vi "RunExperiment2.vi"(0 "object in":refnum<class "Application.lvclass">, 5 "error in (no error)":errorcluster) -> (14 "object out":refnum<class "Application.lvclass">, 15 "Average FPS":dbl, 16 "Waveform Graph":dbl[](graph), 17 "Finished":bool, 19 "error out":errorcluster)   [LabVIEW 2024, in "Application.lvclass"]
uses:
  Application.lvclass
  ExperimentSeries2_class/ExperimentSeries2.lvclass
  Experiment2_class/Experiment2.lvclass
  AD2_SDK_class/AD2_SDK.lvclass
  Hamamatsu_class/Hamamatsu.lvclass
  Application.lvclass/Application.ctl
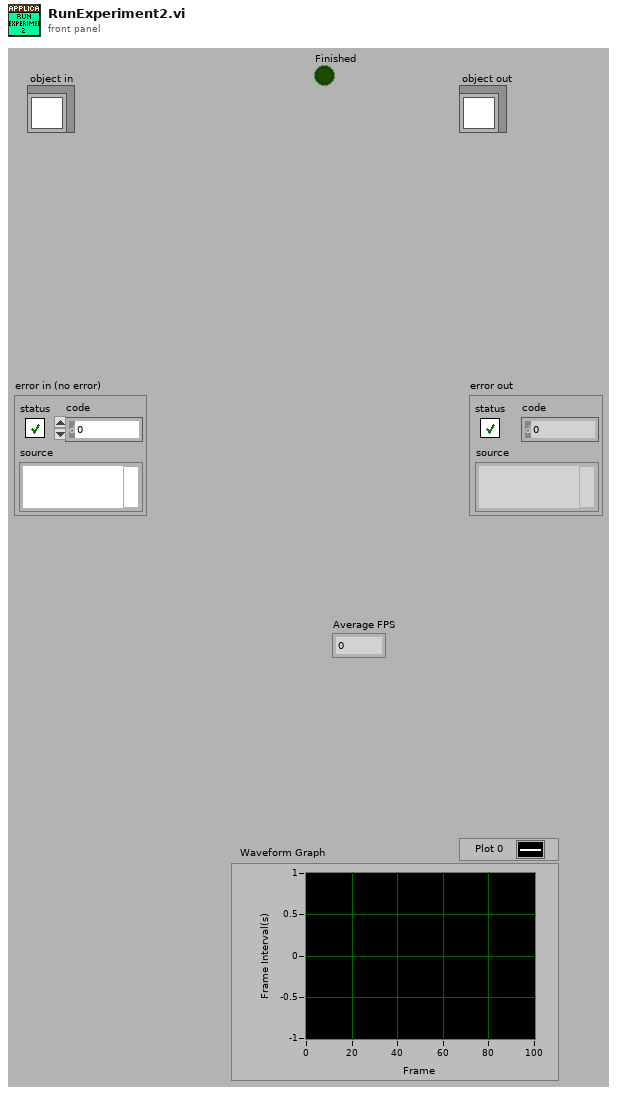
[diagram p1: front panel]
types:
  T1 = typedef "AD2_WFG_SDK.lvclass/WFG.ctl" = cluster{"Running":bool, "Ch1":T2, "Ch2":T2, "SyncronizeState":enum16{"Independent", "Ch1Master", "Ch2Master"}}
  T2 = typedef "AD2_WFG_SDK.lvclass/WFGCh.ctl" = cluster{"idxChannel":i32, "Settings out of range":bool, "Carrier":cluster{"Frequency (Hz)":dbl, "Amplitude (V)":dbl, "Offset(V)":dbl, "Symmetry(%) ":dbl, "Phase(Deg)":dbl, "Function":u16, "Enable":bool}, "Trigger":cluster{"secRun(0=Cont)":dbl, "secWait":dbl, "cRepeat(0=inf)":i32, "Repeat Trigger":bool, "TrigrSrc":T3}, "FM Mod":cluster{"Frequency (Hz)":dbl, "Amplitude (%)":dbl, "Offset(V)":dbl, "Symmetry(%) ":dbl, "Phase(Deg)":dbl, "Function 2":u16, "Enable":bool}}
  T3 = typedef "AD2_SDK.lvclass/AD2TriggerSources.ctl" = enum8{"trigrsrcNone", "trigsrcPC", "trigsrcDetectorAnalogIn", "trigsrcDetectorDigitalIn", "trigsrcAnalogIn", "trigsrcDigitalIn", "trigsrcDigitalOut", "trigsrcAnalogOut1", "trigsrcAnalogOut2", "trigsrcAnalogOut3", "trigsrcAnalogOut4", "trigsrcExternal1", "trigsrcExternal2", "trigsrcExternal3", "trigsrcExternal4", ""}
  T4 = typedef "AD2_DO_SDK.lvclass/DOTrigger.ctl" = cluster{"secRun(0=Cont)":dbl, "secWait":dbl, "cRepeat(0=inf)":i32, "Repeat Trigger":bool, "TrigrSrc":T3}
  T5 = cluster{"DO Trigger":T4, "ClockSettings":cluster{"Frequency":dbl, "Enable":bool, "IdleState":enum16{"Initial", "Low", "High", "Z"}}[]}
  T6 = cluster{"Frequency":dbl, "Enable":bool, "IdleState":enum16{"Initial", "Low", "High", "Z"}}[]
  T7 = cluster{"Master Pulse Settings":cluster{"Mode":u32, "Source":u32, "Interval":dbl, "Burst":u32}, "Capture mode":i32, "Frames":i32, "Dcam Trigger Source":i32, "External Options":cluster{"Polarity":i32, "Delay":dbl}, "ExposureTime(ms)":dbl}
  T8 = cluster{"Flush Flowrate":dbl, "flush volume (ul)":dbl, "WaitAfterFlush":dbl}
  T9 = typedef "Hamamatsu.lvclass/SubRegionLimits.ctl" = cluster{"H Offset":cluster{"Value":i32, "Limits":T10}, "V Offset":cluster{"Value":i32, "Limits":T10}, "H Size":cluster{"Value":i32, "Limits":T10}, "V Size":cluster{"Value":i32, "Limits":T10}}
  T10 = typedef "LVMinMaxIncTypeDef.ctl" = cluster{"Minimum":dbl, "Maximum":dbl, "Increment":dbl}
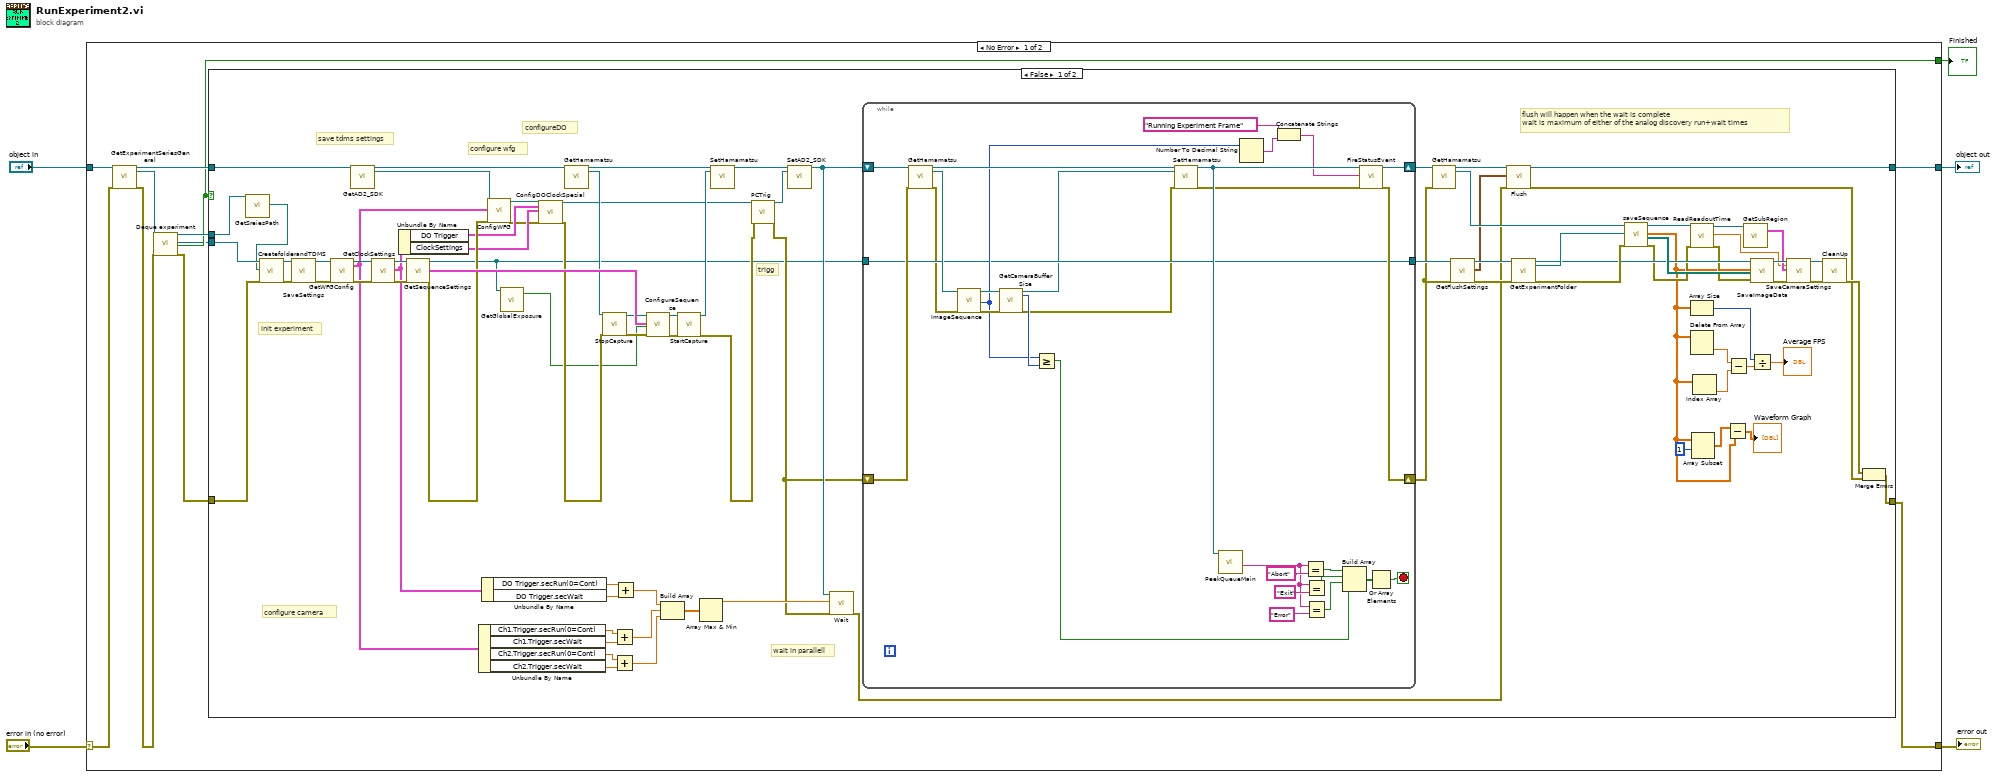
[diagram p0: block diagram]
diagram:
  n1 = case shown="No Error" "error in (no error)" {
    selector: "error in (no error)" -> [w12 w135]
    tunnel: [w8 w135] -> w4
    tunnel: [w16 w134] -> w2
    tunnel: "object in" -> [w15 w134]
    tunnel: [w7 _] -> w1
    frame No Error {
      n2 = call-dynamic "GetExperimentSeriesGeneral.vi"("object in"=w15, "error in (no error)"=w12) -> ("object out"=w14:refnum<class "Application.lvclass">, "ExperimentSeriesGeneral"=w13:refnum<class "ExperimentSeries2.lvclass">, "error out"=w11:errorcluster)  [unwired: 15 in]
      n3 = call-dynamic "Deque experiment.vi"("object in"=w13, "error in (no error)"=w11) -> ("object out"=w10:refnum<class "ExperimentSeries2.lvclass">, "Experiment2"=w6:refnum<class "Experiment2.lvclass">, "timed out?"=w7:bool, "error out"=w9:errorcluster)  [unwired: 14 in]
      n4 = case shown="False" w7 {
        tunnel: [w60 w133] -> w16
        tunnel: w14 -> [w102 w133]
        tunnel: w9 -> [w88 w132]
        tunnel: w10 -> [w72 _]
        tunnel: [w74 w132] -> w8
        tunnel: w6 -> [w99 _]
        frame False {
          # "wait in parallell"
          # "flush will happen when the wait is complete\nwait is maximum of either of the analog discovery run+wait times"
          # "init experiment"
          # "save tdms settings"
          # "trigg"
          # "configureDO"
          # "configure wfg"
          # "configure camera"
          n5 = call-dynamic "GetSreiesPath.vi"("object in"=w72) -> ("SeriesPath"=w71:path)  [unwired: 16 in, 2 out]
          n6 = call "CreatefolderandTDMS.vi"("object in"=w99, "Experiment Series"=w71, "error in (no error)"=w88) -> ("object out"=w98:refnum<class "Experiment2.lvclass">, "error out"=w97:errorcluster)  [unwired: 15 in]
          n7 = call-dynamic "SaveSettings.vi"("object in"=w98, "error in (no error)"=w97) -> ("object out"=w96:refnum<class "Experiment2.lvclass">, "error out"=w95:errorcluster)  [unwired: 16 in]
          n8 = call-dynamic "GetWFGConfig.vi"("object in"=w96, "error in (no error)"=w95) -> ("object out"=w65:refnum<class "Experiment2.lvclass">, "WFGConfig"=w34:T1, "error out"=w67:errorcluster)  [unwired: 15 in]
          n9 = call-dynamic "GetAD2_SDK.vi"("object in"=w102) -> ("object out"=w100:refnum<class "Application.lvclass">, "AD2_SDK"=w101:refnum<class "AD2_SDK.lvclass">)  [unwired: 16 in, 1 out]
          n10 = call-dynamic "GetClockSettings.vi"("object in"=w65, "error in (no error)"=w67) -> ("object out"=w64:refnum<class "Experiment2.lvclass">, "DOClockSettings"=w19:T5, "error out"=w66:errorcluster)  [unwired: 15 in]
          n11 = Unbundle By Name(w19) -> ("DO Trigger"=w63:T4, "ClockSettings"=w62:T6)
          n12 = call-dynamic "GetSequenceSettings.vi"("object in"=w64, "error in (no error)"=w66) -> ("object out"=w18:refnum<class "Experiment2.lvclass">, "Sequence Settings"=w93:T7, "error out"=w84:errorcluster)  [unwired: 15 in]
          n13 = Unbundle By Name(w34) -> ("Ch1.Trigger.secRun(0=Cont)"=w30:dbl, "Ch1.Trigger.secWait"=w31:dbl, "Ch2.Trigger.secRun(0=Cont)"=w29:dbl, "Ch2.Trigger.secWait"=w28:dbl)
          n14 = Unbundle By Name(w19) -> ("DO Trigger.secRun(0=Cont)"=w33:dbl, "DO Trigger.secWait"=w32:dbl)
          n15 = call-dynamic "ConfigWFG.vi"("object in"=w101, "Config(var)"=w34, "error in (no error)"=w84) -> ("object out"=w68:refnum<class "AD2_SDK.lvclass">, "error out"=w61:errorcluster)  [unwired: 15 in]
          n16 = call-dynamic "GetGlobalExposure.vi"("object in"=w18) -> ("GlobalExposure"=w17:bool)  [unwired: 16 in, 2 out]
          n17 = call-dynamic "ConfigDOClockSpezial.vi"("object in"=w68, "DO Trigger"=w63, "ClockSettings"=w62, "error in (no error)"=w61) -> ("object out"=w69:refnum<class "AD2_SDK.lvclass">, "error out"=w70:errorcluster)  [unwired: 14 in]
          n18 = call-dynamic "GetHamamatsu.vi"("object in"=w100) -> ("object out"=w94:refnum<class "Application.lvclass">, "Hamamatsu"=w87:refnum<class "Hamamatsu.lvclass">)  [unwired: 16 in, 1 out]
          n19 = call-dynamic "StopCapture.vi"("object in"=w87, "error in (no error)"=w70) -> ("object out"=w91:refnum<class "Hamamatsu.lvclass">, "error out"=w90:errorcluster)  [unwired: 16 in]
          n20 = Add(x=w30, y=w31) -> (x+y=w26:dbl)
          n21 = Add(x=w29, y=w28) -> (x+y=w25:dbl)
          n22 = Add(x=w33, y=w32) -> (x+y=w27:dbl)
          n23 = call-dynamic "ConfigureSequence.vi"("object in"=w91, "Sequence Settings"=w93, "globalshutter"=w17, "error in (no error)"=w90) -> ("object out"=w92:refnum<class "Hamamatsu.lvclass">, "error out"=w89:errorcluster)  [unwired: 14 in]
          n24 = Build Array(w27, w26, w25) -> (w24:dbl[])
          n25 = call-dynamic "StartCapture.vi"("object in"=w92, "error in (no error)"=w89) -> ("object out"=w86:refnum<class "Hamamatsu.lvclass">, "error out"=w82:errorcluster)  [unwired: 16 in]
          n26 = Array Max & Min(array=w24) -> (max value=w23:dbl)  [unwired: 3 out]
          n27 = call-dynamic "SetHamamatsu.vi"("object in"=w94, "Hamamatsu"=w86) -> ("object out"=w85:refnum<class "Application.lvclass">)  [unwired: 16 in, 1 out]
          n28 = call-dynamic "PCTrig.vi"("object in"=w69, "error in (no error)"=w82) -> ("object out"=w83:refnum<class "AD2_SDK.lvclass">, "error out"=w20:errorcluster)  [unwired: 16 in]
          n29 = call-dynamic "SetAD2_SDK.vi"("object in"=w85, "AD2_SDK"=w83) -> ("object out"=w22:refnum<class "Application.lvclass">)  [unwired: 16 in, 1 out]
          n30 = call-dynamic "Wait.vi"("object in"=w22, "Wait (s)"=w23, "error in (no error)"=w20) -> ("error out"=w21:errorcluster)  [unwired: 15 in, 1 out]
          n31 = while {
            shift-right: [w120] -> w49
            shift-left: w22 -> [w122]
            shift-right: [w113] -> w45
            shift-left: w20 -> [w115]
            tunnel: w18 -> [w107]
            tunnel: [w107] -> w80
            stop <- w117 stop-if-true
            n32 = call-dynamic "GetHamamatsu.vi"("object in"=w122, "error in (no error)"=w115) -> ("object out"=w131:refnum<class "Application.lvclass">, "Hamamatsu"=w112:refnum<class "Hamamatsu.lvclass">, "error out"=w104:errorcluster)  [unwired: 15 in]
            n33 = call-dynamic "ImageSequence.vi"("object in"=w112, "error in (no error)"=w104) -> ("object out"=w110:refnum<class "Hamamatsu.lvclass">, "Frame Count"=w108:i32, "error out"=w111:errorcluster)  [unwired: 14 in, 1 out]
            n34 = call-dynamic "GetCameraBufferSize.vi"("object in"=w110, "error in (no error)"=w111) -> ("object out"=w105:refnum<class "Hamamatsu.lvclass">, "CameraBufferSize"=w109:i32, "error out"=w106:errorcluster)  [unwired: 15 in]
            n35 = Greater Or Equal?(x=w108, y=w109) -> (x >= y?=w103:bool)
            n36 = call-dynamic "SetHamamatsu.vi"("object in"=w131, "Hamamatsu"=w105, "error in (no error)"=w106) -> ("object out"=w121:refnum<class "Application.lvclass">, "error out"=w114:errorcluster)  [unwired: 15 in]
            n37 = call-dynamic "PeekQueueMain.vi"("object in"=w121) -> ("Message"=w123:string)  [unwired: 15 in, 3 out]
            n38 = Number To Decimal String(number=w108) -> (decimal integer string=w116:string)  [unwired: 1 in]
            n39 = Concatenate Strings("Running Experiment Frame" ("string"), w116) -> (w118:string)
            n40 = Equal?(x=w123, y="Abort") -> (x = y?=w126:bool)
            n41 = Equal?(x=w123, y="Exit") -> (x = y?=w125:bool)
            n42 = Equal?(x=w123, y="Error") -> (x = y?=w127:bool)
            n43 = Build Array(w126, w125, w127, w103) -> (w124:bool[])
            n44 = call-dynamic "FireStatusEvent.vi"("object in"=w121, "Status"=w118, "error in (no error)"=w114) -> ("object out"=w120:refnum<class "Application.lvclass">, "error out"=w113:errorcluster)  [unwired: 15 in]
            n45 = Or Array Elements(Boolean array=w124) -> (logical OR=w117:bool)
          }
          n46 = call-dynamic "GetHamamatsu.vi"("object in"=w49, "error in (no error)"=w45) -> ("object out"=w48:refnum<class "Application.lvclass">, "Hamamatsu"=w81:refnum<class "Hamamatsu.lvclass">)  [unwired: 15 in, 1 out]
          n47 = call-dynamic "GetFlushSettings.vi"("object in"=w80, "error in (no error)"=w45) -> ("object out"=w47:refnum<class "Experiment2.lvclass">, "Flush Settings"=w44:T8, "error out"=w46:errorcluster)  [unwired: 15 in]
          n48 = call-dynamic "Flush.vi"("object in"=w48, "Flush Settings"=w44, "error in (no error)"=w21) -> ("object out"=w60:refnum<class "Application.lvclass">, "error out"=w75:errorcluster)  [unwired: 15 in]
          n49 = call-dynamic "GetExperimentFolder.vi"("object in"=w47, "error in (no error)"=w46) -> ("object out"=w73:refnum<class "Experiment2.lvclass">, "ExperimentFolder"=w79:path, "error out"=w78:errorcluster)  [unwired: 15 in]
          n50 = call-dynamic "saveSequence.vi"("object in"=w81, "folder path"=w79, "error in (no error)"=w78) -> ("object out"=w55:refnum<class "Hamamatsu.lvclass">, "Timestamps"=w37:dbl[], "Filenames"=w77:path[], "error out"=w54:errorcluster)  [unwired: 13 in]
          n51 = call-dynamic "ReadReadoutTime.vi"("object in"=w55, "error in (no error)"=w54) -> ("object out"=w52:refnum<class "Hamamatsu.lvclass">, "ReadoutTime"=w50:dbl, "error out"=w53:errorcluster)  [unwired: 15 in]
          n52 = Array Size(array=w37) -> (size(s)=w41:i32)
          n53 = Delete From Array(array=w37) -> (deleted portion=w42:dbl)  [unwired: 2 in, 1 out]
          n54 = Array Subset(array=w37, index=1) -> (w38:dbl[])  [unwired: 1 in]
          n55 = Index Array(array=w37) -> (element=w43:dbl)  [unwired: 1 in]
          n56 = Subtract(x=w38, y=w37) -> (x-y=→"Waveform Graph":dbl[])
          n57 = Subtract(x=w42, y=w43) -> (x-y=w40:dbl)
          n58 = call-dynamic "GetSubRegion.vi"("object in"=w52) -> ("Sub Region"=w51:T9)  [unwired: 16 in, 2 out]
          n59 = call-dynamic "SaveImageData.vi"("object in"=w73, "Timestamps"=w37, "Filenames"=w77, "error in (no error)"=w53) -> ("object out"=w59:refnum<class "Experiment2.lvclass">, "error out"=w57:errorcluster)  [unwired: 14 in]
          n60 = Divide(x=w41, y=w40) -> (x/y=→"Average FPS":dbl)
          n61 = call-dynamic "SaveCameraSettings.vi"("object in"=w59, "ReadoutTime"=w50, "Sub Region"=w51, "error in (no error)"=w57) -> ("object out"=w58:refnum<class "Experiment2.lvclass">, "error out"=w56:errorcluster)  [unwired: 14 in]
          n62 = call-dynamic "CleanUp.vi"("object in"=w58, "error in (no error)"=w56) -> ("error out"=w76:errorcluster)  [unwired: 16 in, 1 out]
          n63 = Merge Errors(w76, w75) -> (w74:errorcluster)
        }
        frame True {
        }
      }
    }
    frame Error {
    }
  }
  "error out" <- w4
  "object out" <- w2
  "Finished" <- w1
